vi "校准设置页.vi"() -> ()   [LabVIEW 2016, in "斯坦道总氮.lvlib"]
uses:
  <vilib>/Analysis/6fits.llb/Curve Fitting Criteria.ctl
  <vilib>/Analysis/NI_AALPro.lvlib
panel:
  in  "跨度核查":bool
  in  "零点核查":bool
  in  "标样核查":bool
  in  "标样校准":bool
  in  "空白校准":bool
  in  "校准导入":bool
  in  "辅助计算":bool
  in  "曲线模型":T1={"标液浓度1"=0.0, "测量吸光度1"=0.0, "样品1启用"=FALSE, "标液浓度2"=0.0, "测量吸光度2"=0.0, "样品2启用"=FALSE, "标液浓度3"=0.0, "测量吸光度3"=0.0, "样品3启用"=FALSE, "标液浓度4"=0.0, "测量吸光度4"=0.0, "样品4启用"=FALSE, "标液浓度5"=0.0, "测量吸光度5"=0.0, "样品5启用"=FALSE, "模型"=enum."线性", "精度"=4.0, "XY图"=[], "拟合公式"="", "r^2"=0.0, "标样一校准时间"=timestamp(0 s since 1904-01-01), "标样二校准时间"=timestamp(0 s since 1904-01-01), "标样三校准时间"=timestamp(0 s since 1904-01-01), "标样四校准时间"=timestamp(0 s since 1904-01-01), "标样五校准时间"=timestamp(0 s since 1904-01-01), "二次方程"={"c"=0.0, "x"=0.0, "x^2"=0.0}, "标定时间"=timestamp(0 s since 1904-01-01)} {"标定时间" format="%<%m/%d/%y %H:%M:%S>T"; "标样五校准时间" format="%<%m/%d/%y %H:%M:%S>T"; "标样四校准时间" format="%<%m/%d/%y %H:%M:%S>T"; "标样三校准时间" format="%<%m/%d/%y %H:%M:%S>T"; "标样二校准时间" format="%<%m/%d/%y %H:%M:%S>T"; "标样一校准时间" format="%<%m/%d/%y %H:%M:%S>T"; "r^2" format="%.7f"; "测量吸光度5" format="%#.6f"; "测量吸光度4" format="%#.6f"; "测量吸光度3" format="%#.6f"; "测量吸光度2" format="%#.6f"; "测量吸光度1" format="%#.6f"}
  in  "测量模式":enum16{"水样测量", "零点核查", "跨度核查", "标样核查", "加标回收"}(ring)
  in  "参数下拉列表":u16(ring)
  in  "量程下拉列表":enum16{"低量程", "高量程"}(ring)
  # "校准时间"
  # "标液浓度"
  # "吸光值显示"
  # "标液一"
  # "标液二"
  # "标液三"
  # "零点"
  # "跨度"
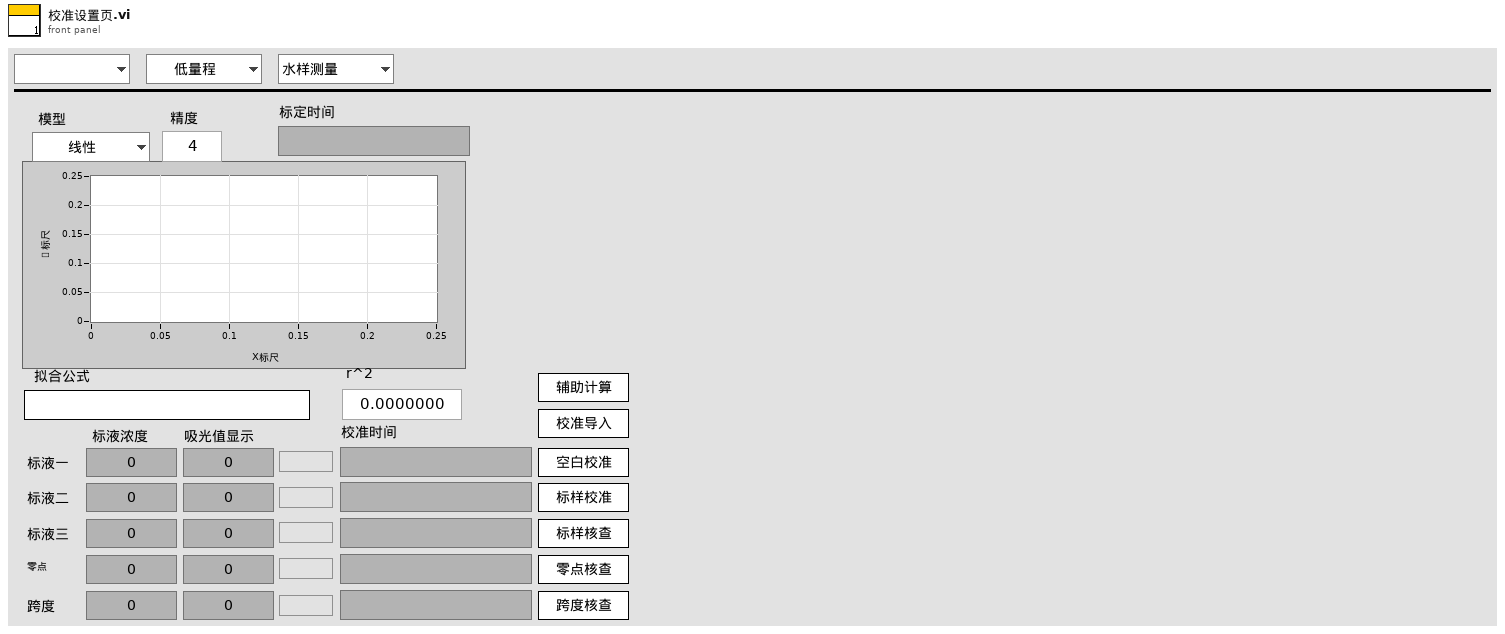
[diagram p1: front panel]
types:
  T1 = cluster{"标液浓度1":dbl, "测量吸光度1":dbl, "样品1启用":bool, "标液浓度2":dbl, "测量吸光度2":dbl, "样品2启用":bool, "标液浓度3":dbl, "测量吸光度3":dbl, "样品3启用":bool, "标液浓度4":dbl, "测量吸光度4":dbl, "样品4启用":bool, "标液浓度5":dbl, "测量吸光度5":dbl, "样品5启用":bool, "模型":enum32{"线性", "多项式"}, "精度":dbl, "XY图":cluster{"X Values":dbl[], "Y Values":dbl[]}[], "拟合公式":string, "r^2":dbl, "标样一校准时间":timestamp, "标样二校准时间":timestamp, "标样三校准时间":timestamp, "标样四校准时间":timestamp, "标样五校准时间":timestamp, "二次方程":cluster{"c":dbl, "x":dbl, "x^2":dbl}, "标定时间":timestamp}
  T2 = typedef "LVStringsAndValuesArrayTypeDef_U16.ctl" = cluster{"String":string, "Value":u16}[]
  T3 = enum8{"Enabled", "Disabled", "Disabled and Grayed Out"}
  T4 = enum16{"启动测量", "标样核查", "零点核查", "跨度核查", "空白测试", "平行样测试", "加标回收", "空白校准", "标样校准", "初始化（清洗）", "停止测试", "仪器重启", "校时", "模式设置", "测量间隔设置"}
  T5 = cluster{"站号":u16, "量程切换":enum32{"H", "L", "AUTO"}, "控制命令":enum16{"启动测量", "标样核查", "零点核查", "跨度核查", "空白测试", "平行样测试", "加标回收", "空白校准", "标样校准", "初始化（清洗）", "停止测试", "仪器重启", "校时", "模式设置", "测量间隔设置"}, "模式设置":enum16{"待机", "连续模式", "周期模式", "定点模式", "受控模式", "手动模式"}, "测量间隔":u16}
  T6 = cluster{"标液浓度1":dbl, "测量吸光度1":dbl, "样品1启用":bool, "标液浓度2":dbl, "测量吸光度2":dbl, "样品2启用":bool, "标液浓度3":dbl, "测量吸光度3":dbl, "样品3启用":bool, "标液浓度4":dbl, "测量吸光度4":dbl, "样品4启用":bool, "标液浓度5":dbl, "测量吸光度5":dbl, "样品5启用":bool, "模型":enum32{"线性", "多项式"}, "精度":dbl, "XY图":cluster{"X Values":dbl[], "Y Values":dbl[]}[], "拟合公式":string, "r^2":dbl, "标样一校准时间":timestamp, "标样二校准时间":timestamp, "标样三校准时间":timestamp, "标样四校准时间":timestamp, "标样五校准时间":timestamp, "二次方程":cluster{"c":dbl, "x":dbl, "x^2":dbl}, "标定时间":timestamp}[][]
  T7 = enum16{"Left Button", "Center Button", "Right Button", "Window Close"}
  T8 = typedef "NI_AALPro.lvlib/Curve Fitting Criteria.ctl" = u16
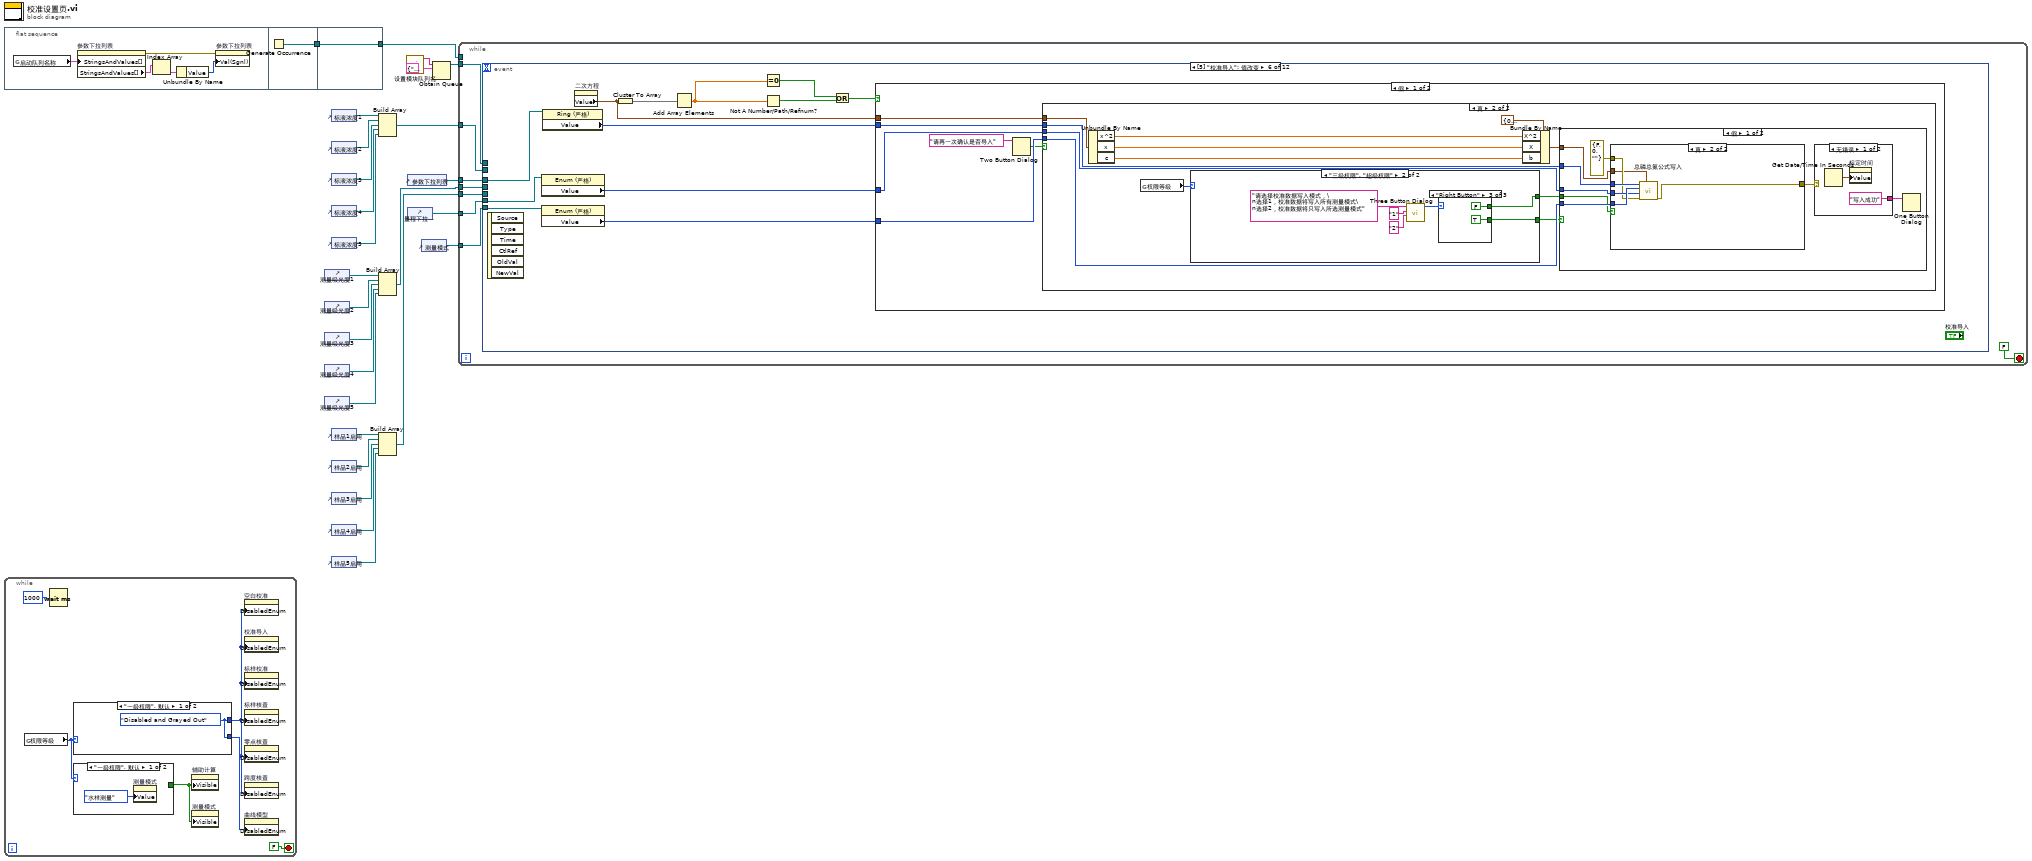
[diagram p0: block diagram]
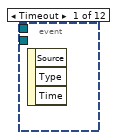
[diagram p2: hidden frame]
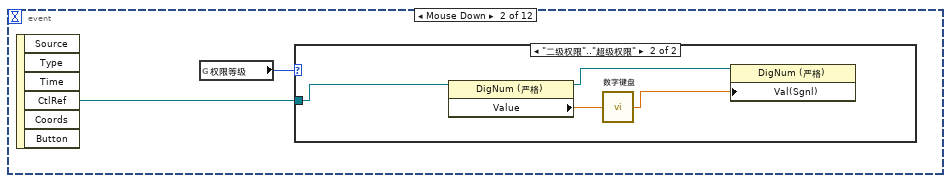
[diagram p3: hidden frame]
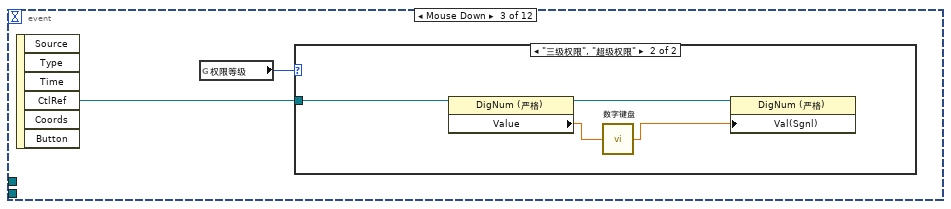
[diagram p5: hidden frame]
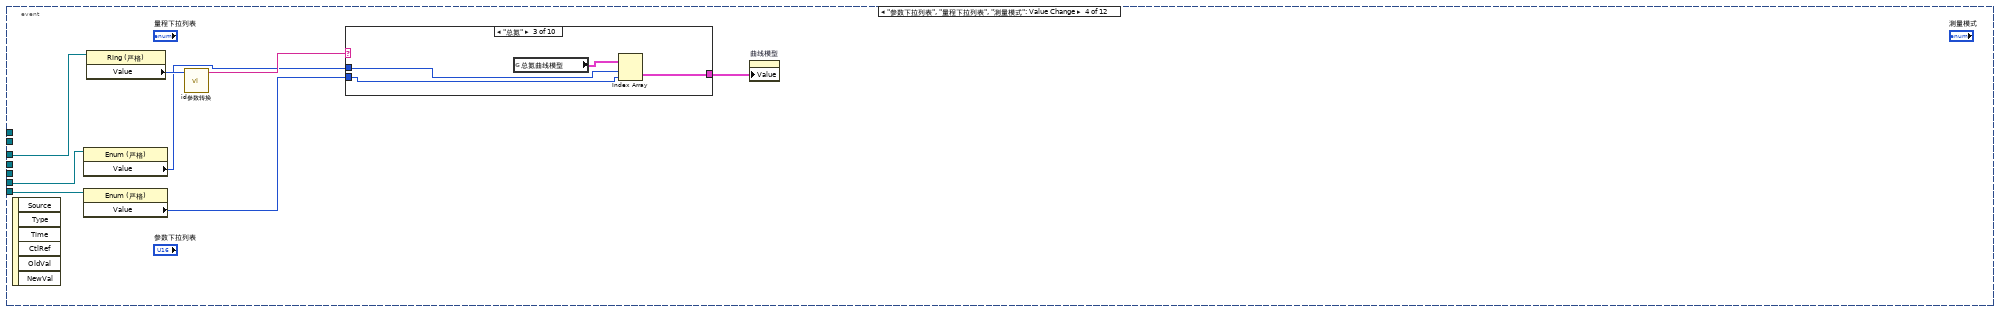
[diagram p7: hidden frame]
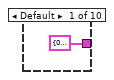
[diagram p8: hidden frame]
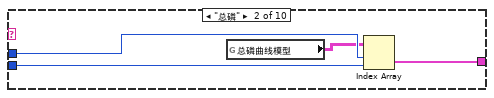
[diagram p9: hidden frame]
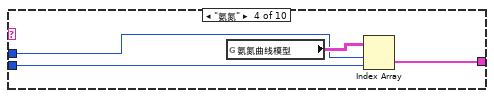
[diagram p10: hidden frame]
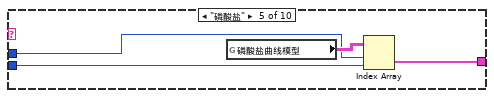
[diagram p11: hidden frame]
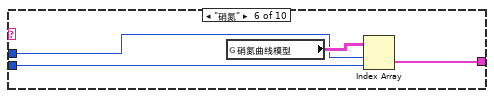
[diagram p12: hidden frame]
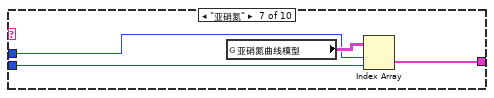
[diagram p13: hidden frame]
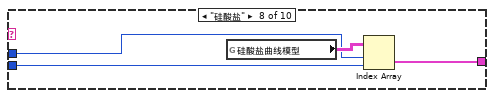
[diagram p14: hidden frame]
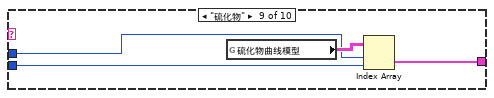
[diagram p15: hidden frame]
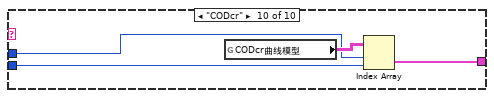
[diagram p16: hidden frame]
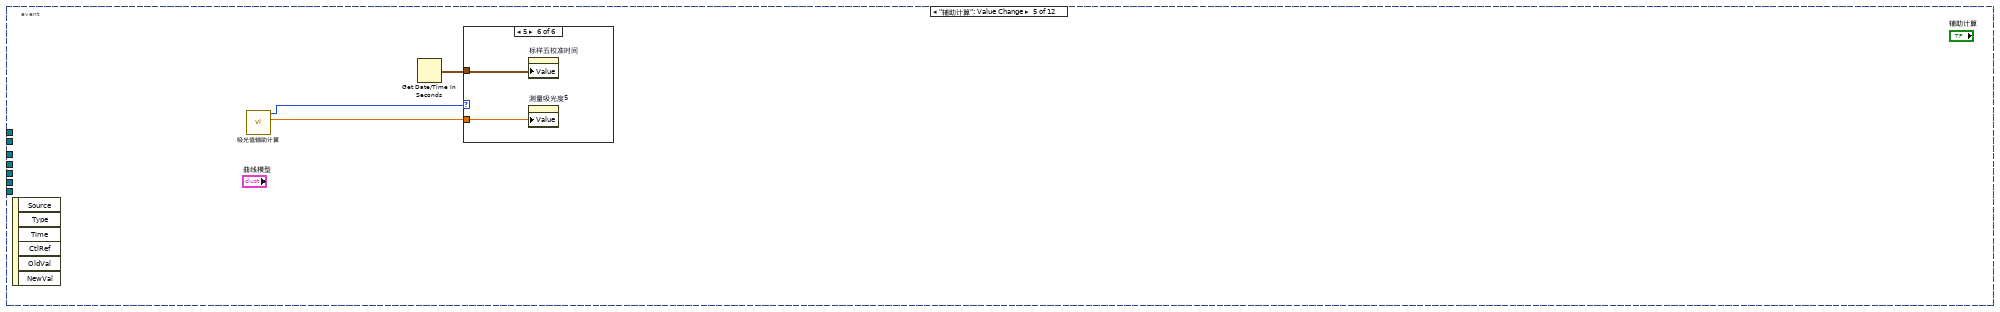
[diagram p17: hidden frame]
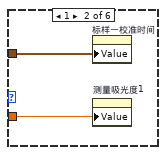
[diagram p19: hidden frame]
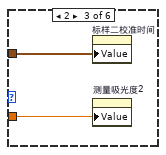
[diagram p20: hidden frame]
diagram:
  n1 = flat-sequence {
    tunnel: [w32] -> w26
    tunnel: [w33] -> w25
    tunnel: w26 -> [w33]
    frame #0 {
      n2 = global read "总磷总氮断电保存全局变量.vi" "启动队列名称"() -> (w27:cluster{"String":string, "Value":u16}[])
      n3 = property on="参数下拉列表" class="Ring (严格)"("StringsAndValues[]"=w27) -> (error out=w30:errorcluster, "StringsAndValues[]"=w28:T2)  [unwired: 2 in, 1 out]
      n4 = Index Array(array=w28) -> (element=w29:cluster{"String":string, "Value":u16})  [unwired: 1 in]
      n5 = Unbundle By Name(w29) -> ("Value"=w31:u16)
      n6 = property on="参数下拉列表" class="Ring (严格)"(error in=w30, "Val(Sgnl)"=w31) -> ()  [unwired: 1 in, 2 out]
    }
    frame #1 {
      n7 = Generate Occurrence() -> (w32:refnum<k4>)
    }
    frame #2 {
    }
  }
  n8 = while {
    stop <- FALSE stop-if-true
    n9 = global read "VAR总磷总氮全局变量.vi" "权限等级"() -> (w35:enum16{"一级权限", "二级权限", "三级权限", "超级权限"})
    n10 = Wait (ms)(milliseconds to wait=u32 1000 ("等待时间（毫秒）")) -> ()  [unwired: 1 out]
    n11 = case shown="\"一级权限\", 默认" w35 {
      tunnel: [w42 w43] -> w37
      tunnel: [w42 w43] -> w36
      frame "一级权限", Default {
        w42 = T3."Disabled and Grayed Out" ("禁用")
      }
      frame "二级权限".."超级权限" {
        w43 = T3."Enabled" ("禁用")
      }
    }
    n12 = case shown="\"一级权限\", 默认" w35 {
      tunnel: [_ TRUE ("可见")] -> w34
      frame "一级权限", Default {
        n13 = property on="测量模式" class="Enum (严格)"("Value"=enum16{"水样测量", "零点核查", "跨度核查", "标样核查", "加标回收"}."水样测量" ("测量模式")) -> ()  [unwired: 2 in, 2 out]
      }
      frame "三级权限", "超级权限" {
      }
    }
    n14 = property on="辅助计算" class="Bool"("Visible"=w34) -> ()  [unwired: 2 in, 2 out]
    n15 = property on="测量模式" class="Enum (严格)"("Visible"=w34) -> ()  [unwired: 2 in, 2 out]
    n16 = property on="空白校准" class="Bool"("DisabledEnum"=w36) -> ()  [unwired: 2 in, 2 out]
    n17 = property on="校准导入" class="Bool"("DisabledEnum"=w36) -> ()  [unwired: 2 in, 2 out]
    n18 = property on="标样校准" class="Bool"("DisabledEnum"=w36) -> ()  [unwired: 2 in, 2 out]
    n19 = property on="标样核查" class="Bool"("DisabledEnum"=w36) -> ()  [unwired: 2 in, 2 out]
    n20 = property on="零点核查" class="Bool"("DisabledEnum"=w36) -> ()  [unwired: 2 in, 2 out]
    n21 = property on="跨度核查" class="Bool"("DisabledEnum"=w36) -> ()  [unwired: 2 in, 2 out]
    n22 = property on="曲线模型" class="Clust (严格)"("DisabledEnum"=w37) -> ()  [unwired: 2 in, 2 out]
  }
  n23 = control-ref of="测量吸光度1"() -> (w13:refnum<vi>)
  n24 = control-ref of="测量吸光度2"() -> (w14:refnum<vi>)
  n25 = control-ref of="测量吸光度3"() -> (w15:refnum<vi>)
  n26 = control-ref of="测量吸光度4"() -> (w16:refnum<vi>)
  n27 = control-ref of="测量吸光度5"() -> (w17:refnum<vi>)
  n28 = control-ref of="标液浓度1"() -> (w11:refnum<vi>)
  n29 = control-ref of="标液浓度2"() -> (w10:refnum<vi>)
  n30 = control-ref of="标液浓度3"() -> (w9:refnum<vi>)
  n31 = control-ref of="标液浓度4"() -> (w8:refnum<vi>)
  n32 = control-ref of="标液浓度5"() -> (w7:refnum<vi>)
  n33 = control-ref of="样品1启用"() -> (w23:refnum<vi>)
  n34 = control-ref of="样品2启用"() -> (w22:refnum<vi>)
  n35 = control-ref of="样品3启用"() -> (w21:refnum<vi>)
  n36 = control-ref of="样品4启用"() -> (w20:refnum<vi>)
  n37 = control-ref of="样品5启用"() -> (w19:refnum<vi>)
  n38 = Build Array(w11, w10, w9, w8, w7) -> (w6:refnum<vi>[])
  n39 = Build Array(w13, w14, w15, w16, w17) -> (w12:refnum<vi>[])
  n40 = Build Array(w23, w22, w21, w20, w19) -> (w18:refnum<vi>[])
  n41 = call "设置模块队列名.vi"() -> ("Msg"=w2:string)  [unwired: 5 in]
  n42 = control-ref of="参数下拉列表"() -> (w24:refnum<vi>)
  n43 = control-ref of="量程下拉列表"() -> (w4:refnum<vi>)
  n44 = control-ref of="测量模式"() -> (w5:refnum<vi>)
  n45 = Obtain Queue(name (unnamed)=w2, element data type=cluster{"命令":string, "data":variant} {"命令"="", "data"=variant}) -> (queue out=w1:refnum<queue>)  [unwired: 3 in, 2 out]
  n46 = while {
    tunnel: w25 -> [_]
    tunnel: w24 -> [w50]
    tunnel: w18 -> [w49]
    tunnel: w12 -> [w48]
    tunnel: w6 -> [w47]
    tunnel: w5 -> [w46]
    tunnel: w4 -> [w45]
    tunnel: w1 -> [w44]
    stop <- FALSE stop-if-true
    n47 = event shown="[5] \"校准导入\": 值改变" {
      selector: _ -> [_ _ _ _ _ _ _ _ _ _ _ _]
      dyn-events: _ -> [_ _ _ _ _ _ _ _ _ _ _ _]
      timeout: _ -> [_ _ _ _ _ _ _ _ _ _ _ _]
      tunnel: w50 -> [_ _ _ w70 _ w133 w197 w288 w301 w314 w327 w340]
      tunnel: w49 -> [_ _ _ _ _ _ w201 _ _ _ _ _]
      tunnel: w48 -> [_ _ _ _ _ _ w200 _ _ _ _ _]
      tunnel: w47 -> [_ _ _ _ _ _ w199 _ _ _ _ _]
      tunnel: w46 -> [_ _ _ w68 _ w131 w195 _ _ _ _ _]
      tunnel: w45 -> [_ _ _ w67 _ w129 w193 w283 w296 w309 w322 w335]
      tunnel: w44 -> [_ _ _ _ _ _ _ w291 w304 w317 w330 w343]
      event Timeout {
        n48 = event-data() -> ()  [unwired: 1 in, 3 out]
      }
      event "曲线模型.标液浓度1", "曲线模型.标液浓度2", "曲线模型.标液浓度3", "曲线模型.标液浓度4", "曲线模型.标液浓度5", "曲线模型.精度": Mouse Down {
        n49 = event-data() -> ("CtlRef"=w53:refnum<vi>)  [unwired: 1 in, 5 out]
        n50 = global read "VAR总磷总氮全局变量.vi" "权限等级"() -> (w52:enum16{"一级权限", "二级权限", "三级权限", "超级权限"})
        n51 = case shown="\"二级权限\"..\"超级权限\"" w52 {
          tunnel: w53 -> [_ w57]
          frame "一级权限", Default {
          }
          frame "二级权限".."超级权限" {
            n52 = property class="DigNum (严格)"(reference=w57) -> (reference out=w55:refnum<vi>, "Value"=w56:dbl)  [unwired: 1 in, 1 out]
            n53 = call "数字键盘.vi"("OldNumber"=w56) -> ("NewNumber"=w54:dbl)
            n54 = property class="DigNum (严格)"(reference=w55, "Val(Sgnl)"=w54) -> ()  [unwired: 1 in, 2 out]
          }
        }
      }
      event "曲线模型.测量吸光度1", "曲线模型.测量吸光度2", "曲线模型.测量吸光度3", "曲线模型.测量吸光度4", "曲线模型.测量吸光度5": Mouse Down {
        n55 = event-data() -> ("CtlRef"=w59:refnum<vi>)  [unwired: 1 in, 5 out]
        n56 = global read "VAR总磷总氮全局变量.vi" "权限等级"() -> (w58:enum16{"一级权限", "二级权限", "三级权限", "超级权限"})
        n57 = case shown="\"三级权限\", \"超级权限\"" w58 {
          tunnel: w59 -> [_ w63]
          frame "一级权限", Default {
          }
          frame "三级权限", "超级权限" {
            n58 = property class="DigNum (严格)"(reference=w63) -> (reference out=w61:refnum<vi>, "Value"=w62:dbl)  [unwired: 1 in, 1 out]
            n59 = call "数字键盘.vi"("OldNumber"=w62) -> ("NewNumber"=w60:dbl)
            n60 = property class="DigNum (严格)"(reference=w61, "Val(Sgnl)"=w60) -> ()  [unwired: 1 in, 2 out]
          }
        }
      }
      event "参数下拉列表", "量程下拉列表", "测量模式": Value Change {
        n61 = event-data() -> ()  [unwired: 1 in, 6 out]
        n62 = property class="Enum (严格)"(reference=w67) -> ("Value"=w66:enum16{"低量程", "高量程"})  [unwired: 1 in, 2 out]
        n63 = property class="Enum (严格)"(reference=w68) -> ("Value"=w65:enum16{"水样测量", "零点核查", "跨度核查", "标样核查", "加标回收"})  [unwired: 1 in, 2 out]
        n64 = property class="Ring (严格)"(reference=w70) -> ("Value"=w71:u16)  [unwired: 1 in, 2 out]
        n65 = call "id参数转换.vi"("id"=w71) -> ("table输出"=w69:string)  [unwired: 9 in, 1 out]
        n66 = case shown="\"总氮\"" w69 {
          tunnel: w65 -> [_ w75 w80 w82 w86 w90 w94 w98 w102 w106]
          tunnel: w66 -> [_ w76 w79 w83 w87 w91 w95 w99 w103 w107]
          tunnel: [T1 {"标液浓度1"=0.0, "测量吸光度1"=0.0, "样品1启用"=FALSE, "标液浓度2"=0.0, "测量吸光度2"=0.0, "样品2启用"=FALSE, "标液浓度3"=0.0, "测量吸光度3"=0.0, "样品3启用"=FALSE, "标液浓度4"=0.0, "测量吸光度4"=0.0, "样品4启用"=FALSE, "标液浓度5"=0.0, "测量吸光度5"=0.0, "样品5启用"=FALSE, "模型"=enum."线性", "精度"=0.0, "XY图"=[], "拟合公式"="", "r^2"=0.0, "标样一校准时间"=timestamp(0 s since 1904-01-01), "标样二校准时间"=timestamp(0 s since 1904-01-01), "标样三校准时间"=timestamp(0 s since 1904-01-01), "标样四校准时间"=timestamp(0 s since 1904-01-01), "标样五校准时间"=timestamp(0 s since 1904-01-01), "二次方程"={"c"=0.0, "x"=0.0, "x^2"=0.0}, "标定时间"=timestamp(0 s since 1904-01-01)} ("总磷曲线模型") w73 w77 w81 w85 w89 w93 w97 w101 w105] -> w64
          frame Default {
          }
          frame "总磷" {
            n67 = global read "校准数据全局变量.vi" "总磷曲线模型"() -> (w74:T6)
            n68 = Index Array(array=w74, index (row)=w76, index (col)=w75) -> (element=w73:T1)
          }
          frame "总氮" {
            n69 = global read "校准数据全局变量.vi" "总氮曲线模型"() -> (w78:T6)
            n70 = Index Array(array=w78, index (row)=w79, index (col)=w80) -> (element=w77:T1)
          }
          frame "氨氮" {
            n71 = global read "校准数据全局变量.vi" "氨氮曲线模型"() -> (w84:T6)
            n72 = Index Array(array=w84, index (row)=w83, index (col)=w82) -> (element=w81:T1)
          }
          frame "磷酸盐" {
            n73 = global read "校准数据全局变量.vi" "磷酸盐曲线模型"() -> (w88:T6)
            n74 = Index Array(array=w88, index (row)=w87, index (col)=w86) -> (element=w85:T1)
          }
          frame "硝氮" {
            n75 = global read "校准数据全局变量.vi" "硝氮曲线模型"() -> (w92:T6)
            n76 = Index Array(array=w92, index (row)=w91, index (col)=w90) -> (element=w89:T1)
          }
          frame "亚硝氮" {
            n77 = global read "校准数据全局变量.vi" "亚硝氮曲线模型"() -> (w96:T6)
            n78 = Index Array(array=w96, index (row)=w95, index (col)=w94) -> (element=w93:T1)
          }
          frame "硅酸盐" {
            n79 = global read "校准数据全局变量.vi" "硅酸盐曲线模型"() -> (w100:T6)
            n80 = Index Array(array=w100, index (row)=w99, index (col)=w98) -> (element=w97:T1)
          }
          frame "硫化物" {
            n81 = global read "校准数据全局变量.vi" "硫化物曲线模型"() -> (w104:T6)
            n82 = Index Array(array=w104, index (row)=w103, index (col)=w102) -> (element=w101:T1)
          }
          frame "CODcr" {
            n83 = global read "校准数据全局变量.vi" "CODcr曲线模型"() -> (w108:T6)
            n84 = Index Array(array=w108, index (row)=w107, index (col)=w106) -> (element=w105:T1)
          }
        }
        n85 = property on="曲线模型" class="Clust (严格)"("Value"=w64) -> ()  [unwired: 2 in, 2 out]
      }
      event "辅助计算": Value Change {
        n86 = event-data() -> ()  [unwired: 1 in, 6 out]
        n87 = call "吸光值辅助计算.vi"() -> ("X"=w110:dbl, "吸光值导出"=w111:u16)  [unwired: 10 in]
        n88 = Get Date/Time In Seconds() -> (seconds since 1Jan1904=w109:timestamp)
        n89 = case shown="5" w111 {
          tunnel: w110 -> [_ w113 w115 w117 w119 w121]
          tunnel: w109 -> [_ w112 w114 w116 w118 w120]
          frame 0, Default {
          }
          frame 1 {
            n90 = property on="标样一校准时间" class="AbsTime (严格)"("Value"=w112) -> ()  [unwired: 2 in, 2 out]
            n91 = property on="测量吸光度1" class="DigNum (严格)"("Value"=w113) -> ()  [unwired: 2 in, 2 out]
          }
          frame 2 {
            n92 = property on="标样二校准时间" class="AbsTime (严格)"("Value"=w114) -> ()  [unwired: 2 in, 2 out]
            n93 = property on="测量吸光度2" class="DigNum (严格)"("Value"=w115) -> ()  [unwired: 2 in, 2 out]
          }
          frame 3 {
            n94 = property on="标样三校准时间" class="AbsTime (严格)"("Value"=w116) -> ()  [unwired: 2 in, 2 out]
            n95 = property on="测量吸光度3" class="DigNum (严格)"("Value"=w117) -> ()  [unwired: 2 in, 2 out]
          }
          frame 4 {
            n96 = property on="标样四校准时间" class="AbsTime (严格)"("Value"=w118) -> ()  [unwired: 2 in, 2 out]
            n97 = property on="测量吸光度4" class="DigNum (严格)"("Value"=w119) -> ()  [unwired: 2 in, 2 out]
          }
          frame 5 {
            n98 = property on="标样五校准时间" class="AbsTime (严格)"("Value"=w120) -> ()  [unwired: 2 in, 2 out]
            n99 = property on="测量吸光度5" class="DigNum (严格)"("Value"=w121) -> ()  [unwired: 2 in, 2 out]
          }
        }
      }
      event "校准导入": Value Change {
        n100 = event-data() -> ()  [unwired: 1 in, 6 out]
        n101 = property class="Enum (严格)"(reference=w129) -> ("Value"=w128:enum16{"低量程", "高量程"})  [unwired: 1 in, 2 out]
        n102 = property class="Enum (严格)"(reference=w131) -> ("Value"=w130:enum16{"水样测量", "零点核查", "跨度核查", "标样核查", "加标回收"})  [unwired: 1 in, 2 out]
        n103 = property class="Ring (严格)"(reference=w133) -> ("Value"=w132:u16)  [unwired: 1 in, 2 out]
        n104 = property on="二次方程" class="Clust (严格)"() -> ("Value"=w127:cluster{"c":dbl, "x":dbl, "x^2":dbl})  [unwired: 2 in, 2 out]
        n105 = Cluster To Array(cluster=w127) -> (array=w126:dbl[])
        n106 = Add Array Elements(numeric array=w126) -> (sum=w125:dbl)
        n107 = Equal To 0?(x=w125) -> (x = 0?=w123:bool)
        n108 = Not A Number/Path/Refnum?(number/path/refnum=w125) -> (NaN/Path/Refnum?=w124:bool)
        n109 = Or(x=w123, y=w124) -> (x .or. y?=w122:bool)
        n110 = case shown="假" w122 {
          tunnel: w132 -> [w139 _]
          tunnel: w130 -> [w138 _]
          tunnel: w128 -> [w137 _]
          tunnel: w127 -> [w134 _]
          frame False {
            n111 = Two Button Dialog(message="请再一次确认是否导入" ("消息")) -> (T button?=w135:bool)  [unwired: 2 in]
            n112 = case shown="真" w135 {
              tunnel: w139 -> [_ w146]
              tunnel: w138 -> [_ w145]
              tunnel: w137 -> [_ w144]
              tunnel: w134 -> [_ w143]
              frame False {
              }
              frame True {
                n113 = Unbundle By Name(w143) -> ("x^2"=w149:dbl, "x"=w148:dbl, "c"=w147:dbl)
                n114 = global read "VAR总磷总氮全局变量.vi" "权限等级"() -> (w142:enum16{"一级权限", "二级权限", "三级权限", "超级权限"})
                n115 = case shown="\"三级权限\", \"超级权限\"" w142 {
                  tunnel: [FALSE w183] -> w141
                  tunnel: [_ w182] -> w140
                  frame "一级权限", Default {
                  }
                  frame "三级权限", "超级权限" {
                    n116 = call <vilib>:"Three Button Dialog.vi"("Center Button Text (\"No\")"="2" ("Center Button Text (\"No\")"), "Left Button Text (\"Yes\")"="1" ("Left Button Text (\"Yes\")"), "message"="请选择校准数据写入模式，\n选择1，校准数据将写入所有测量模式\n选择2，校准数据将只写入所选测量模式") -> ("Which Button?"=w184:T7)  [unwired: 8 in]
                    n117 = case shown="\"Right Button\"" w184 {
                      tunnel: [FALSE TRUE FALSE] -> w183
                      tunnel: [_ _ TRUE] -> w182
                      frame "Left Button", Default {
                      }
                      frame "Center Button" {
                      }
                      frame "Right Button" {
                      }
                    }
                  }
                }
                n118 = Bundle By Name(cluster=cluster{"X^2":dbl, "X":dbl, "b":dbl} {"X^2"=0.0, "X"=0.0, "b"=0.0} ("公式"), "X^2"=w149, "X"=w148, "b"=w147) -> (w150:cluster{"X^2":dbl, "X":dbl, "b":dbl})
                n119 = case shown="假" w140 {
                  tunnel: w150 -> [w159 _]
                  tunnel: w146 -> [w158 _]
                  tunnel: w145 -> [w157 _]
                  tunnel: w144 -> [w156 _]
                  tunnel: w141 -> [w152 _]
                  frame False {
                    n120 = case shown="真" w152 {
                      tunnel: w159 -> [w166 w172]
                      tunnel: w158 -> [w165 w177]
                      tunnel: w157 -> [w164 w176]
                      tunnel: w156 -> [w163 w175]
                      tunnel: [w162 w174] -> w154
                      tunnel: errorcluster {"status"=FALSE, "code"=0, "source"=""} ("error out") -> [w161 w173]
                      frame False {
                        n121 = for {
                          N: 5 -> [_]
                          tunnel: w166 -> [w171]
                          tunnel: w165 -> [w170]
                          tunnel: w164 -> [_]
                          tunnel: w163 -> [w169]
                          shift-right: [w168] -> w162
                          shift-left: w161 -> [_]
                          i -> [w167]
                          n122 = call "总磷总氮公式写入.vi"("公式"=w171, "量程"=w169, "测量模式"=w167, "测量参数"=w170) -> ("error out"=w168:errorcluster)  [unwired: 7 in]
                        }
                      }
                      frame True {
                        n123 = call "总磷总氮公式写入.vi"("公式"=w172, "error in (no error)"=w173, "量程"=w175, "测量模式"=w176, "测量参数"=w177) -> ("error out"=w174:errorcluster)  [unwired: 6 in]
                      }
                    }
                    n124 = case shown="无错误" w154 {
                      tunnel: ["写入成功" "写入失败"] -> w155
                      frame No Error {
                        n125 = Get Date/Time In Seconds() -> (seconds since 1Jan1904=w178:timestamp)
                        n126 = property on="标定时间" class="AbsTime (严格)"("Value"=w178) -> ()  [unwired: 2 in, 2 out]
                      }
                      frame Error {
                      }
                    }
                    n127 = One Button Dialog(message=w155) -> ()  [unwired: 1 in, 1 out]
                  }
                  frame True {
                  }
                }
              }
            }
          }
          frame True {
            n128 = One Button Dialog(message="校准数据异常，请重新校准！" ("消息")) -> ()  [unwired: 1 in, 1 out]
          }
        }
      }
      event "曲线模型": Value Change {
        n129 = event-data() -> ()  [unwired: 1 in, 6 out]
        n130 = flat-sequence {
          tunnel: w201 -> [w221]
          tunnel: w200 -> [w219]
          tunnel: w199 -> [w217]
          tunnel: [w204] -> w198
          tunnel: w197 -> [w204]
          tunnel: [w203] -> w196
          tunnel: w195 -> [w203]
          tunnel: [w202] -> w194
          tunnel: w193 -> [w202]
          tunnel: w198 -> [w235]
          tunnel: w196 -> [w231]
          tunnel: w194 -> [w229]
          frame #0 {
            w213 = T8 0 items=["最小二乘", "最小绝对残差", "Bisquare"] ("method")
            n131 = for {
              tunnel: w221 -> [w227] mode=indexing
              tunnel: [w226] -> w220 mode=indexing
              tunnel: w219 -> [w225] mode=indexing
              tunnel: [w224] -> w218 mode=indexing
              tunnel: w217 -> [w223] mode=indexing
              tunnel: [w222] -> w216 mode=indexing
              n132 = property class="DigNum (严格)"(reference=w223) -> ("Value"=w222:dbl)  [unwired: 1 in, 2 out]
              n133 = property class="DigNum (严格)"(reference=w225) -> ("Value"=w224:dbl)  [unwired: 1 in, 2 out]
              n134 = property class="Bool (严格)"(reference=w227) -> ("Value"=w226:bool)  [unwired: 1 in, 2 out]
            }
            n135 = property on="模型" class="Enum (严格)"() -> ("Value"=w215:enum32{"线性", "多项式"})  [unwired: 2 in, 2 out]
            n136 = property on="精度" class="DigNum (严格)"() -> ("Value"=w214:dbl)  [unwired: 2 in, 2 out]
            n137 = call "线性公式.vi"("精度"=w214, "模型"=w215, "method"=w213, "启用"=w220, "监测浓度"=w218, "标液浓度"=w216) -> ("Polynomial Coefficients 2"=w209:dbl[], "XY图"=w210:cluster{"X Values":dbl[], "Y Values":dbl[]}[], "r^2"=w211:dbl, "拟合方程"=w212:string)  [unwired: 2 in]
            n138 = property on="拟合公式" class="Str"("Value"=w212) -> ()  [unwired: 2 in, 2 out]
            n139 = property on="r^2" class="DigNum (严格)"("Value"=w211) -> ()  [unwired: 2 in, 2 out]
            n140 = property on="XY图" class="XYGraph (严格)"("Value"=w210) -> ()  [unwired: 2 in, 2 out]
            n141 = Index Array(array=w209) -> (element #1=w208:dbl, element #2=w207:dbl, element #3=w206:dbl)  [unwired: 3 in]
            n142 = Bundle("slope"=w208, "slope"=w207, "slope"=w206) -> (w205:cluster{"slope":dbl, "slope":dbl, "slope":dbl})  [unwired: 1 in]
            n143 = property on="二次方程" class="Clust (严格)"("Value"=w205) -> ()  [unwired: 2 in, 2 out]
          }
          frame #1 {
            n144 = property class="Enum (严格)"(reference=w229) -> ("Value"=w228:enum16{"低量程", "高量程"})  [unwired: 1 in, 2 out]
            n145 = property class="Enum (严格)"(reference=w231) -> ("Value"=w230:enum16{"水样测量", "零点核查", "跨度核查", "标样核查", "加标回收"})  [unwired: 1 in, 2 out]
            n146 = property class="Ring (严格)"(reference=w235) -> ("Value"=w234:u16)  [unwired: 1 in, 2 out]
            n147 = call "id参数转换.vi"("id"=w234) -> ("table输出"=w233:string)  [unwired: 9 in, 1 out]
            n148 = property on="曲线模型" class="Clust (严格)"() -> ("Value"=w232:T1)  [unwired: 2 in, 2 out]
            n149 = case shown="默认" w233 {
              tunnel: w232 -> [_ w240 w245 w247 w251 w256 w261 w266 w271 w277]
              tunnel: w230 -> [_ w238 w244 w248 w252 w257 w262 w267 w272 w278]
              tunnel: w228 -> [_ w239 w243 w249 w253 w258 w263 w268 w273 w279]
              frame Default {
              }
              frame "总磷" {
                n150 = global read "校准数据全局变量.vi" "总磷曲线模型"() -> (w236:T6)
                n151 = Replace Array Subset(array=w236, new element=w240, index (row)=w239, index (col)=w238) -> (w237:T6)
                n152 = global write "校准数据全局变量.vi" "总磷曲线模型"(w237) -> ()
              }
              frame "总氮" {
                n153 = global read "校准数据全局变量.vi" "总氮曲线模型"() -> (w242:T6)
                n154 = Replace Array Subset(array=w242, new element=w245, index (row)=w243, index (col)=w244) -> (w241:T6)
                n155 = global write "校准数据全局变量.vi" "总氮曲线模型"(w241) -> ()
              }
              frame "氨氮" {
                n156 = global read "校准数据全局变量.vi" "氨氮曲线模型"() -> (w250:T6)
                n157 = Replace Array Subset(array=w250, new element=w247, index (row)=w249, index (col)=w248) -> (w246:T6)
                n158 = global write "校准数据全局变量.vi" "氨氮曲线模型"(w246) -> ()
              }
              frame "磷酸盐" {
                n159 = global read "校准数据全局变量.vi" "磷酸盐曲线模型"() -> (w255:T6)
                n160 = Replace Array Subset(array=w255, new element=w251, index (row)=w253, index (col)=w252) -> (w254:T6)
                n161 = global write "校准数据全局变量.vi" "磷酸盐曲线模型"(w254) -> ()
              }
              frame "硝氮" {
                n162 = global read "校准数据全局变量.vi" "硝氮曲线模型"() -> (w260:T6)
                n163 = Replace Array Subset(array=w260, new element=w256, index (row)=w258, index (col)=w257) -> (w259:T6)
                n164 = global write "校准数据全局变量.vi" "硝氮曲线模型"(w259) -> ()
              }
              frame "亚硝氮" {
                n165 = global read "校准数据全局变量.vi" "亚硝氮曲线模型"() -> (w265:T6)
                n166 = Replace Array Subset(array=w265, new element=w261, index (row)=w263, index (col)=w262) -> (w264:T6)
                n167 = global write "校准数据全局变量.vi" "亚硝氮曲线模型"(w264) -> ()
              }
              frame "硅酸盐" {
                n168 = global read "校准数据全局变量.vi" "硅酸盐曲线模型"() -> (w270:T6)
                n169 = Replace Array Subset(array=w270, new element=w266, index (row)=w268, index (col)=w267) -> (w269:T6)
                n170 = global write "校准数据全局变量.vi" "硅酸盐曲线模型"(w269) -> ()
              }
              frame "硫化物" {
                n171 = global read "校准数据全局变量.vi" "硫化物曲线模型"() -> (w275:T6)
                n172 = Replace Array Subset(array=w275, new element=w271, index (row)=w273, index (col)=w272) -> (w274:T6)
                n173 = global write "校准数据全局变量.vi" "硫化物曲线模型"(w274) -> ()
              }
              frame "CODcr" {
                n174 = global read "校准数据全局变量.vi" "CODcr曲线模型"() -> (w280:T6)
                n175 = Replace Array Subset(array=w280, new element=w277, index (row)=w279, index (col)=w278) -> (w276:T6)
                n176 = global write "校准数据全局变量.vi" "CODcr曲线模型"(w276) -> ()
              }
            }
          }
          frame #2 {
            n177 = call "校准数据写入配置文件.vi"() -> ()  [unwired: 11 in, 1 out]
          }
        }
      }
      event "空白校准": Value Change {
        n178 = event-data() -> ()  [unwired: 1 in, 6 out]
        n179 = property class="Enum (严格)"(reference=w283) -> ("Value"=w282:enum16{"低量程", "高量程"})  [unwired: 1 in, 2 out]
        n180 = property class="Ring (严格)"(reference=w288) -> ("Value"=w285:u16)  [unwired: 1 in, 2 out]
        n181 = case shown="\"低量程\", 默认" w282 {
          tunnel: [enum32{"H", "L", "AUTO"}."L" ("量程切换") enum32{"H", "L", "AUTO"}."H" ("量程切换")] -> w281
          frame "低量程", Default {
          }
          frame "高量程" {
          }
        }
        n182 = Flush Queue(queue=w291) -> (queue out=w289:refnum<queue>)  [unwired: 1 in, 2 out]
        n183 = Bundle By Name(cluster=T5 {"站号"=1, "量程切换"=enum."AUTO", "控制命令"=enum."启动测量", "模式设置"=enum."待机", "测量间隔"=0} ("参数"), "站号"=w285, "控制命令"=T4."空白校准", "量程切换"=w281) -> (w286:T5)
        n184 = call "总磷总氮启动命令.vi"("参数"=w286) -> ("启动命令"=w290:cluster{"命令":string, "data":variant})  [unwired: 10 in]
        n185 = Enqueue Element(queue=w289, element=w290) -> ()  [unwired: 2 in, 3 out]
      }
      event "标样校准": Value Change {
        n186 = event-data() -> ()  [unwired: 1 in, 6 out]
        n187 = property class="Enum (严格)"(reference=w296) -> ("Value"=w295:enum16{"低量程", "高量程"})  [unwired: 1 in, 2 out]
        n188 = property class="Ring (严格)"(reference=w301) -> ("Value"=w298:u16)  [unwired: 1 in, 2 out]
        n189 = case shown="\"低量程\", 默认" w295 {
          tunnel: [enum32{"H", "L", "AUTO"}."L" ("量程切换") enum32{"H", "L", "AUTO"}."H" ("量程切换")] -> w294
          frame "低量程", Default {
          }
          frame "高量程" {
          }
        }
        n190 = Flush Queue(queue=w304) -> (queue out=w302:refnum<queue>)  [unwired: 1 in, 2 out]
        n191 = Bundle By Name(cluster=T5 {"站号"=1, "量程切换"=enum."AUTO", "控制命令"=enum."启动测量", "模式设置"=enum."待机", "测量间隔"=0} ("参数"), "站号"=w298, "控制命令"=T4."标样校准", "量程切换"=w294) -> (w299:T5)
        n192 = call "总磷总氮启动命令.vi"("参数"=w299) -> ("启动命令"=w303:cluster{"命令":string, "data":variant})  [unwired: 10 in]
        n193 = Enqueue Element(queue=w302, element=w303) -> ()  [unwired: 2 in, 3 out]
      }
      event "标样核查": Value Change {
        n194 = event-data() -> ()  [unwired: 1 in, 6 out]
        n195 = property class="Enum (严格)"(reference=w309) -> ("Value"=w308:enum16{"低量程", "高量程"})  [unwired: 1 in, 2 out]
        n196 = property class="Ring (严格)"(reference=w314) -> ("Value"=w311:u16)  [unwired: 1 in, 2 out]
        n197 = case shown="\"低量程\", 默认" w308 {
          tunnel: [enum32{"H", "L", "AUTO"}."L" ("量程切换") enum32{"H", "L", "AUTO"}."H" ("量程切换")] -> w307
          frame "低量程", Default {
          }
          frame "高量程" {
          }
        }
        n198 = Flush Queue(queue=w317) -> (queue out=w315:refnum<queue>)  [unwired: 1 in, 2 out]
        n199 = Bundle By Name(cluster=T5 {"站号"=1, "量程切换"=enum."AUTO", "控制命令"=enum."启动测量", "模式设置"=enum."待机", "测量间隔"=0} ("参数"), "站号"=w311, "控制命令"=T4."标样核查", "量程切换"=w307) -> (w312:T5)
        n200 = call "总磷总氮启动命令.vi"("参数"=w312) -> ("启动命令"=w316:cluster{"命令":string, "data":variant})  [unwired: 10 in]
        n201 = Enqueue Element(queue=w315, element=w316) -> ()  [unwired: 2 in, 3 out]
      }
      event "零点核查": Value Change {
        n202 = event-data() -> ()  [unwired: 1 in, 6 out]
        n203 = property class="Enum (严格)"(reference=w322) -> ("Value"=w321:enum16{"低量程", "高量程"})  [unwired: 1 in, 2 out]
        n204 = property class="Ring (严格)"(reference=w327) -> ("Value"=w324:u16)  [unwired: 1 in, 2 out]
        n205 = case shown="\"低量程\", 默认" w321 {
          tunnel: [enum32{"H", "L", "AUTO"}."L" ("量程切换") enum32{"H", "L", "AUTO"}."H" ("量程切换")] -> w320
          frame "低量程", Default {
          }
          frame "高量程" {
          }
        }
        n206 = Flush Queue(queue=w330) -> (queue out=w328:refnum<queue>)  [unwired: 1 in, 2 out]
        n207 = Bundle By Name(cluster=T5 {"站号"=1, "量程切换"=enum."AUTO", "控制命令"=enum."启动测量", "模式设置"=enum."待机", "测量间隔"=0} ("参数"), "站号"=w324, "控制命令"=T4."零点核查", "量程切换"=w320) -> (w325:T5)
        n208 = call "总磷总氮启动命令.vi"("参数"=w325) -> ("启动命令"=w329:cluster{"命令":string, "data":variant})  [unwired: 10 in]
        n209 = Enqueue Element(queue=w328, element=w329) -> ()  [unwired: 2 in, 3 out]
      }
      event "跨度核查": Value Change {
        n210 = event-data() -> ()  [unwired: 1 in, 6 out]
        n211 = property class="Enum (严格)"(reference=w335) -> ("Value"=w334:enum16{"低量程", "高量程"})  [unwired: 1 in, 2 out]
        n212 = property class="Ring (严格)"(reference=w340) -> ("Value"=w337:u16)  [unwired: 1 in, 2 out]
        n213 = case shown="\"低量程\", 默认" w334 {
          tunnel: [enum32{"H", "L", "AUTO"}."L" ("量程切换") enum32{"H", "L", "AUTO"}."H" ("量程切换")] -> w333
          frame "低量程", Default {
          }
          frame "高量程" {
          }
        }
        n214 = Flush Queue(queue=w343) -> (queue out=w341:refnum<queue>)  [unwired: 1 in, 2 out]
        n215 = Bundle By Name(cluster=T5 {"站号"=1, "量程切换"=enum."AUTO", "控制命令"=enum."启动测量", "模式设置"=enum."待机", "测量间隔"=0} ("参数"), "站号"=w337, "控制命令"=T4."跨度核查", "量程切换"=w333) -> (w338:T5)
        n216 = call "总磷总氮启动命令.vi"("参数"=w338) -> ("启动命令"=w342:cluster{"命令":string, "data":variant})  [unwired: 10 in]
        n217 = Enqueue Element(queue=w341, element=w342) -> ()  [unwired: 2 in, 3 out]
      }
    }
  }
